vi "IsNotARefnum.vi"(11 "MockListImp in":refnum<class "ListImp_RefSpy.lvclass">) -> (2 "Not a Refnum?":bool, 3 "MockListImp out":refnum<class "ListImp_RefSpy.lvclass">)   [LabVIEW 2009, in "ListImp_RefSpy.lvclass"]
uses:
  ListImp_RefSpy.lvclass
  RefnumGlobal.vi
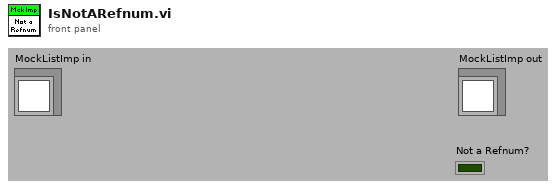
[diagram p1: front panel]
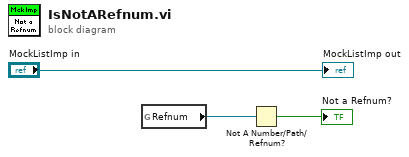
[diagram p0: block diagram]
diagram:
  n1 = global read "RefnumGlobal.vi" "Refnum"() -> (w1:refnum<queue>)
  n2 = Not A Number/Path/Refnum?(number/path/refnum=w1) -> (NaN/Path/Refnum?=→"Not a Refnum?":bool)
  "MockListImp out" <- "MockListImp in"
